vi "Sort.vi"(6 "Variant in":variant, 7 "Shift Pressed?":bool, 8 "error in (no error)":errorcluster, 10 "QD Combo Box Ref":refnum<vi>, 11 "QD Launch VI Ref":refnum<vi>) -> (0 "error out":errorcluster, 4 "Variant out":variant)   [LabVIEW 2017, in "Quick Drop.lvlib"]
doc: "Alphabetizes the elements in a cluster.\n\nDefault Shortcut - [C]"
uses:
  Quick Drop.lvlib
  Toolkit/Toolkit.lvlib
panel:
  in  "Undo Name":string="Sort"
  # "Do not change the connector pane of this VI.\n\nSee the block diagram for directions on how to use this template."
  # "Specify the name of the Undo transaction"
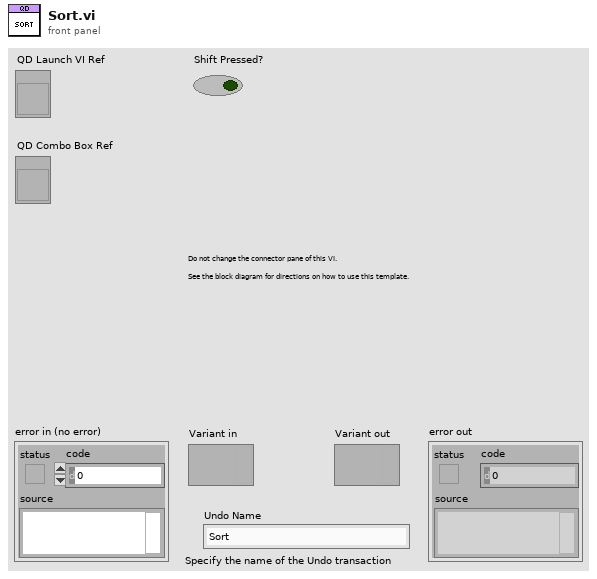
[diagram p1: front panel]
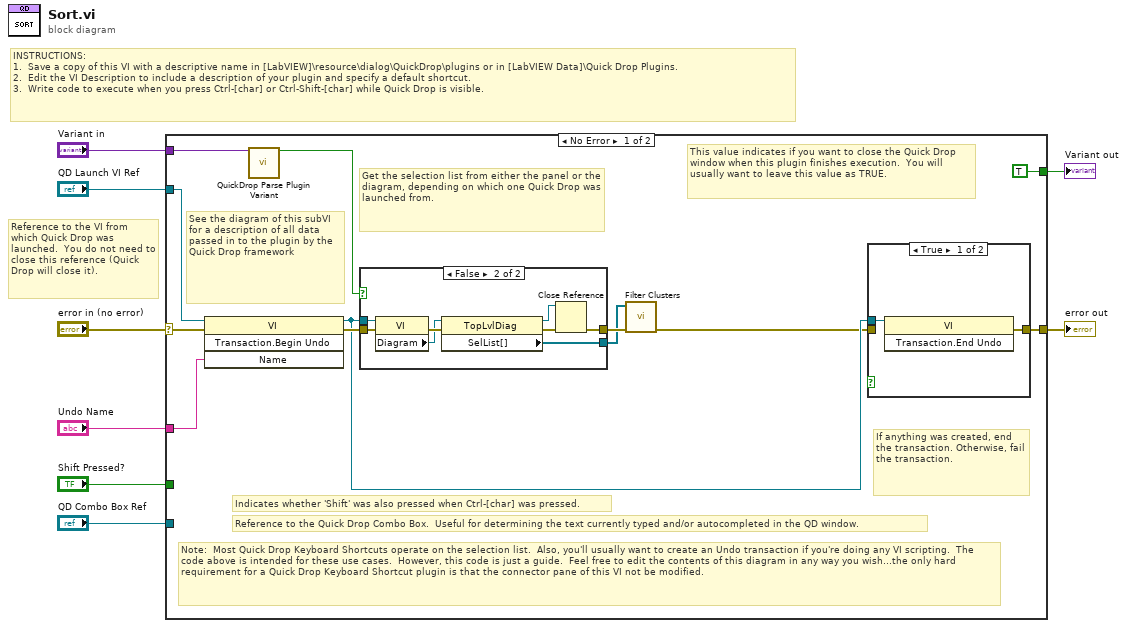
[diagram p0: block diagram]
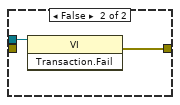
[diagram p2: hidden frame]
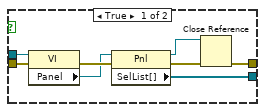
[diagram p3: hidden frame]
diagram:
  # "Reference to the VI from which Quick Drop was launched.  You do not need to close this reference (Quick Drop will close it)."
  # "INSTRUCTIONS:\n1.  Save a copy of this VI with a descriptive name in [LabVIEW]\\resource\\dialog\\QuickDrop\\plugins or in [LabVIEW Data]\\Quick Drop Plugins.\n2.  Edit the VI Description to include a description of your plugin and specify a default shortcut. \n3.  Write code to execute when you press Ctrl-[char] or Ctrl-Shift-[char] while Quick Drop is visible."
  n1 = case shown="No Error" "error in (no error)" {
    selector: "error in (no error)" -> [w19 w41]
    tunnel: [w13 w41] -> w7
    tunnel: "QD Launch VI Ref" -> [w18 _]
    tunnel: "Shift Pressed?" -> [_ _]
    tunnel: "QD Combo Box Ref" -> [_ _]
    tunnel: "Variant in" -> [w20 _]
    tunnel: "Undo Name" -> [w17 _]
    tunnel: [TRUE _] -> w1
    frame No Error {
      # "Note:  Most Quick Drop Keyboard Shortcuts operate on the selection list.  Also, you'll usually want to create an Undo transaction if you're doing any VI scripting.  The code above is intended for these use cases.  However, this code is just a guide.  Feel free to edit the contents of this diagram in any way you wish...the only hard requirement for a Quick Drop Keyboard Shortcut plugin is that the connector pane of this VI not be modified."
      # "Get the selection list from either the panel or the diagram, depending on which one Quick Drop was launched from."
      # "If anything was created, end the transaction. Otherwise, fail the transaction."
      # "This value indicates if you want to close the Quick Drop window when this plugin finishes execution.  You will usually want to leave this value as TRUE."
      # "See the diagram of this subVI for a description of all data passed in to the plugin by the Quick Drop framework"
      # "Reference to the Quick Drop Combo Box.  Useful for determining the text currently typed and/or autocompleted in the QD window."
      # "Indicates whether 'Shift' was also pressed when Ctrl-[char] was pressed."
      n2 = invoke class="VI" method="Transaction.Begin Undo"(reference=w18, error in=w19, "Name"=w17) -> (reference out=w12:refnum<vi>, error out=w14:errorcluster)  [unwired: 1 in, 2 out]
      n3 = call <vilib>:"QuickDrop Parse Plugin Variant.vi"("QDKS Variant in"=w20) -> ("QD Launch VI Panel?"=w15:bool)  [unwired: 12 in, 2 out]
      n4 = case shown="False" w15 {
        tunnel: w14 -> [w32 w40]
        tunnel: w12 -> [w31 w39]
        tunnel: [w26 w34] -> w11
        tunnel: [w25 w33] -> w10
        frame True {
          n5 = property class="VI"(reference=w31, error in=w32) -> (error out=w30:errorcluster, "Panel"=w29:refnum<vi>)  [unwired: 1 out]
          n6 = property class="Pnl"(reference=w29, error in=w30) -> (reference out=w27:refnum<vi>, error out=w28:errorcluster, "SelList[]"=w25:refnum<vi>[])
          n7 = Close Reference(reference=w27, error in (no error)=w28) -> (error out=w26:errorcluster)
        }
        frame False {
          n8 = property class="VI"(reference=w39, error in=w40) -> (error out=w38:errorcluster, "Diagram"=w37:refnum<vi>)  [unwired: 1 out]
          n9 = property class="TopLvlDiag"(reference=w37, error in=w38) -> (reference out=w35:refnum<vi>, error out=w36:errorcluster, "SelList[]"=w33:refnum<vi>[])
          n10 = Close Reference(reference=w35, error in (no error)=w36) -> (error out=w34:errorcluster)
        }
      }
      n11 = call "Filter Clusters.vi"("Error In"=w11, "GObjects"=w10) -> ("Error Out"=w9:errorcluster)  [unwired: 8 in, 1 out]
      n12 = case shown="True" {
        selector: _ -> [_ _]
        tunnel: w12 -> [w21 w23]
        tunnel: [w22 w24] -> w13
        tunnel: w9 -> [_ _]
        frame True {
          n13 = invoke class="VI" method="Transaction.End Undo"(reference=w21) -> (error out=w22:errorcluster)  [unwired: 2 in, 2 out]
        }
        frame False {
          n14 = invoke class="VI" method="Transaction.Fail"(reference=w23) -> (error out=w24:errorcluster)  [unwired: 2 in, 2 out]
        }
      }
    }
    frame Error {
    }
  }
  "error out" <- w7
  "Variant out" <- w1
